vi "WPI_CameraAttributeAsNumber.vi"(7 "Attr Format":string="CameraAttributes::%s::Value", 8 "error in (no error)":errorcluster, 10 "Attr String":string, 11 "Camera Address In":string) -> (0 "error out":errorcluster, 2 "Numeric":dbl, 3 "Camera Address Out":string)   [LabVIEW 2017]
doc: "Returns the raw value of a numeric camera attribute.\n\nThis software is licensed. Open the labview\\readme\\WPI Robotics Library Open Source License.txt file for more information."
uses:
  <vilib>/userdefined/High Color/IMAQdx.ctl
  <resource>/objmgr/imaqdx.rc
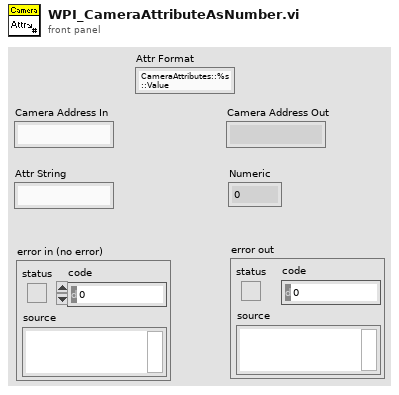
[diagram p1: front panel]
types:
  T1 = typedef "IMAQdx.ctl" = refnum<k21>
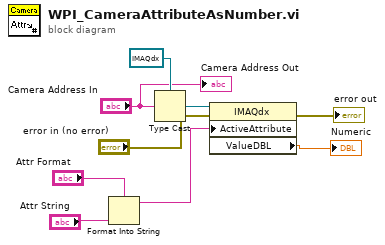
[diagram p0: block diagram]
diagram:
  n1 = Format Into String(format string="Attr Format", "Attr String") -> (resulting string=w5:string)  [unwired: 2 in, 1 out]
  n2 = Type Cast(type=T1 refnum ("Session In"), x="Camera Address In") -> (*(type *) &x=w9:T1)
  n3 = property class="IMAQdx"(reference=w9, error in="error in (no error)", "ActiveAttribute"=w5) -> (error out=→"error out":errorcluster, "ValueDBL"=→"Numeric":dbl)  [unwired: 1 out]
  "Camera Address Out" <- "Camera Address In"
